vi "FT Read GPIO.vi"(0 "handle":u32, 11 "error in (no error)":errorcluster) -> (4 "handle out":u32, 6 "value out":string, 15 "error out":errorcluster)   [LabVIEW 2011, in "libMPSSE.lvlib"]
doc: "FTDI_API FT_STATUS FT_ReadGPIO(FT_HANDLE handle,uint8 *value);"
uses:
  libMPSSE.lvlib
  libMPSSE.dll
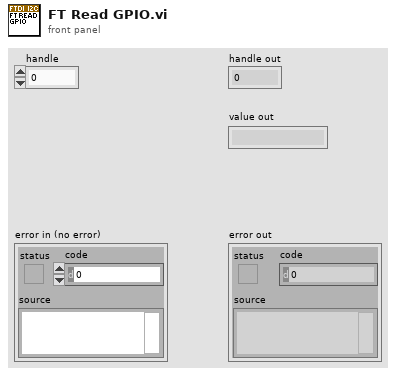
[diagram p1: front panel]
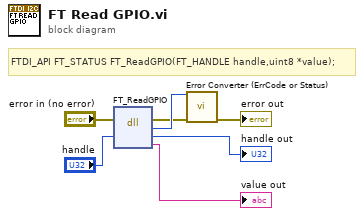
[diagram p0: block diagram]
diagram:
  # "FTDI_API FT_STATUS FT_ReadGPIO(FT_HANDLE handle,uint8 *value);"
  n1 = dll-call lib="D:/Project/HAL_Drivers/I2C/libMPSSE.*" fn="FT_ReadGPIO"(error in="error in (no error)", "handle"="handle") -> (error out=w2:errorcluster, w7:u32, "handle"=→"handle out":u32, "value"=→"value out":string)  [unwired: 3 in, 1 out]
  n2 = call "Error Converter (ErrCode or Status).vi"("error code"=w7, "error in (no error)"=w2) -> ("error out"=→"error out":errorcluster)  [unwired: 13 in]
